vi "Read Variable - Scalar.vi"() -> ()   [LabVIEW 2013, in "GOLPI library.lvlib"]
uses:
  GOLPI library.lvlib
  LV Process.lvlibp
  LV Process.lvlibp/Pipe Handle.ctl
panel:
  in  "variable name":string
  in  "error in":errorcluster
  in  "pipe in":T1
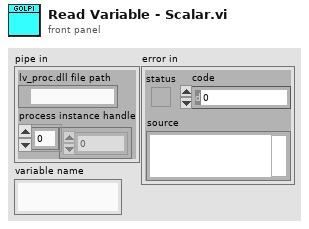
[diagram p1: front panel]
types:
  T1 = typedef "LV Process.lvlibp/Pipe Handle.ctl" = cluster{"lv_proc.dll file path":path, "process instance handle":u32[]}
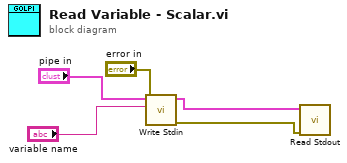
[diagram p0: block diagram]
diagram:
  n1 = call "Write Stdin.vi"("error in"="error in", "write buffer"="variable name", "pipe in"="pipe in") -> ("error out"=w1:errorcluster, "pipe out"=w5:T1)  [unwired: 6 in, 1 out]
  n2 = call "Read Stdout.vi"("error in"=w1, "pipe in"=w5) -> ()  [unwired: 4 in, 6 out]
